vi "PID Turn VISION.vi"(6 "output range":cluster{"output high":dbl, "output low":dbl}={"output high"=100.0, "output low"=-100.0} {"output low" format="%.2f"; "output high" format="%.2f"}, 7 "PID gains":T1={"proportional gain (Kc)"=0.008, "integral time (Ti, min)"=0.0, "derivative time (Td, min)"=0.0013}, 8 "F gain":dbl=0.5, 9 "Gyro":dbl, 10 "Error Tolerance +/- (3)":dbl=2.5, 11 "Setpoint":dbl) -> (2 "Output":dbl, 3 "Angel out":dbl)   [LabVIEW 2015]
uses:
  <vilib>/addons/control/pid/pid.llb/PID Structure.ctl
  <vilib>/addons/control/pid/pid.llb/PID Structure Conversion (DBL).vi
  Code/Robot Global Data.vi
  <vilib>/Rock Robotics/WPI/Utilities/WPI_GetSetVariantRefNum.vi
  <vilib>/addons/control/pid/pid.llb/PID (DBL).vi
  <vilib>/addons/control/pid/NI_PID_pid.lvlib
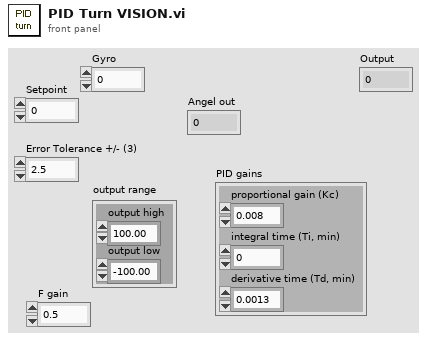
[diagram p1: front panel]
types:
  T1 = cluster{"proportional gain (Kc)":dbl, "integral time (Ti, min)":dbl, "derivative time (Td, min)":dbl}
  T2 = typedef "NI_PID_pid.lvlib/PID Structure.ctl" = u16
  T3 = typedef "WPI_RobotDriveDevRef.ctl" = cluster{"DevStatus":errorcluster, "Motors[]":T4[], "Square Inputs":bool, "Max Output":dbl}
  T4 = typedef "WPI_MotorControlDeviceRef.ctl" = cluster{"DeviceStatus":errorcluster, "Type":T5, "PWM":cluster{"PWM Channel":T6, "DeadBand":T7}, "CAN":cluster{"Device Number":u8, "Control Mode":T8, "Semaphore":T9, "Max Vout":dbl, "TalonSRX Control Mode":T10}, "Invert":bool}
  T5 = typedef "WPI_MotorControlType.ctl" = enum16{"PWM", "CAN", "CANTalonSRX"}
  T6 = typedef "FPGA_DIOPWMChannel.ctl" = enum8{"PWM 0", "PWM 1", "PWM 2", "PWM 3", "PWM 4", "PWM 5", "PWM 6", "PWM 7", "PWM 8", "PWM 9", "PWM MXP 0", "PWM MXP 1", "PWM MXP 2", "PWM MXP 3", "PWM MXP 4", "PWM MXP 5", "PWM MXP 6", "PWM MXP 7", "PWM MXP 8", "PWM MXP 9", "Invalid"}
  T7 = typedef "WPI_PWMDeadband.ctl" = cluster{"Name":string, "maxPositivePwm":i32, "minPositivePwm":i32, "centerPwm":i32, "maxNegativePwm":i32, "minNegativePwm":i32, "angularRange":u16}
  T8 = typedef "WPI_CANJaguar_ControlMode.ctl" = enum8{"Percent VBus", "Current", "Speed", "Position", "Voltage"}
  T9 = typedef "Semaphore RefNum" = refnum<k1>
  T10 = typedef "WPI_CANTalonSRX_APIControlMode.ctl" = enum8{"Percent VBus", "Speed", "Position", "Slave", "Unchanged / Invalid", "Voltage Compensation", "Current", "Motion Profile"}
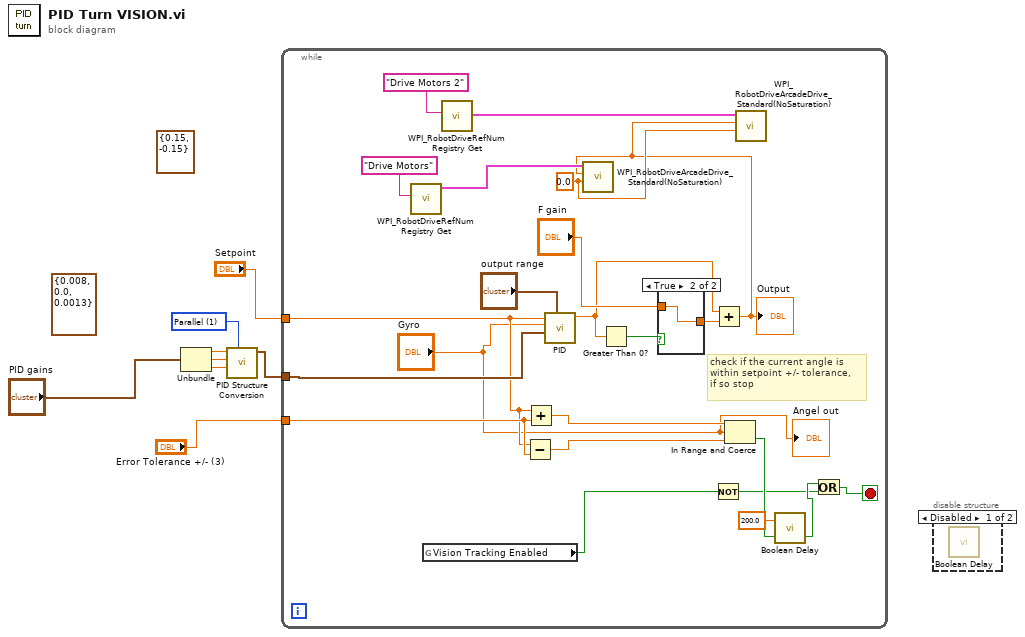
[diagram p0: block diagram]
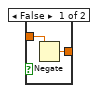
[diagram p3: hidden frame]
diagram:
  (unwired) cluster{"output high":dbl, "output low":dbl} {"output high"=0.15, "output low"=-0.15} ("output range")
  w1 = T2 1 items=["Academic (Standard)", "Parallel", "Series"] ("PID structure")
  (unwired) T1 {"proportional gain (Kc)"=0.008, "integral time (Ti, min)"=0.0, "derivative time (Td, min)"=0.0013} ("PID gains")
  n1 = Unbundle("PID gains") -> ("proportional gain (Kc)"=w6:dbl, "integral time (Ti, min)"=w7:dbl, "derivative time (Td, min)"=w8:dbl)
  n2 = call-poly <vilib>:"PID Structure Conversion.vi"("PID structure"=w1, "derivative"=w8, "integral"=w7, "proportional"=w6) -> ("PID gains"=w4:T1)  [unwired: 7 in]
  n3 = while {
    tunnel: "Setpoint" -> [w12]
    tunnel: w4 -> [w28]
    tunnel: "Error Tolerance +/- (3)" -> [w29]
    stop <- w15 stop-if-true
    w23 = 0.0 ("Y axis value")
    # "check if the current angle is\nwithin setpoint +/- tolerance,\nif so stop"
    n4 = call <vilib>:"WPI_RobotDriveRefNum Registry Get.vi"("refnum name"="Drive Motors") -> ("RobotDriveDevRef"=w24:T3)  [unwired: 1 in, 9 out]
    n5 = global read "Robot Global Data.vi" "Vision Tracking Enabled"() -> (w13:bool)
    n6 = call <vilib>:"WPI_RobotDriveRefNum Registry Get.vi"("refnum name"="Drive Motors 2") -> ("RobotDriveDevRef"=w25:T3)  [unwired: 1 in, 9 out]
    n7 = Subtract(x=w12, y=w29) -> (x-y=w30:dbl)
    n8 = Add(x=w12, y=w29) -> (x+y=w31:dbl)
    n9 = call-poly <vilib>:"PID.vi"("output range"="output range", "PID gains"=w28, "process variable"="Gyro", "setpoint"=w12) -> ("output"=w11:dbl)  [unwired: 6 in, 1 out]
    n10 = Greater Than 0?(x=w11) -> (x > 0?=w27:bool)
    n11 = case shown="True" w27 {
      tunnel: [w32 w34] -> w26
      tunnel: "F gain" -> [w33 w34]
      frame False {
        n12 = Negate(x=w33) -> (-x=w32:dbl)
      }
      frame True {
      }
    }
    n13 = Not(x=w13) -> (.not. x?=w14:bool)
    n14 = Add(x=w11, y=w26) -> (x+y=w22:dbl)
    "Output" <- w22
    n15 = call <vilib>:"WPI_RobotDriveArcadeDrive_Standard(NoSaturation).vi"("Y axis value"=w23, "X axis value"=w22, "RobotDriveDevRef"=w24) -> ()  [unwired: 1 in, 8 out]
    n16 = In Range and Coerce(upper limit=w31, x="Gyro", lower limit=w30) -> (In Range?=w17:bool)  [unwired: 1 out]
    n17 = call <vilib>:"WPI_RobotDriveArcadeDrive_Standard(NoSaturation).vi"("Y axis value"=w23, "X axis value"=w22, "RobotDriveDevRef"=w25) -> ()  [unwired: 1 in, 8 out]
    n18 = call "Boolean Delay.vi"("Input"=w17, "Delay (ms)"=200.0) -> ("Output"=w16:bool)  [unwired: 1 in]
    n19 = Or(x=w16, y=w14) -> (x .or. y?=w15:bool)
    "Angel out" <- "Gyro"
  }
  n20 = disable-structure shown="Disabled" {
    frame Disabled {
      n21 = call "Boolean Delay.vi"() -> ()  [unwired: 3 in, 1 out]
    }
    frame Enabled {
    }
  }
